vi "Configure Polarity.vi"(6 "channel (1)":i32=1 min=1 max=4, 8 "error in (no error)":errorcluster, 10 "Polarity (0: Positive)":T1 items=["Positive", "Negative"], 11 "VISA resource name":refnum<visa-resource-name>) -> (0 "error out":errorcluster, 3 "VISA resource name out":refnum<visa-resource-name>)   [LabVIEW 2019, in "Pulse Rider PG-1000.lvlib"]
doc: "This command set the output polarity.\n\npolarity: the polarity: 'positive' or 'negative'\nchannel: the output channel int from 1 to 4"
uses:
  <instrlib>/LV_PulseRiderPG1000/Pulse Rider PG-1000.lvlib
  <instrlib>/LV_PulseRiderPG1000/Public/Configure/Pulse/Polarity.ctl
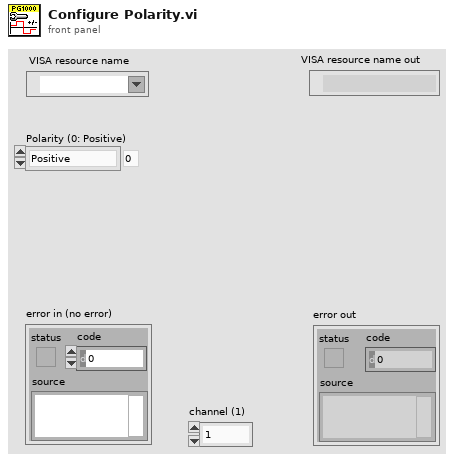
[diagram p1: front panel]
types:
  T1 = typedef "Pulse Rider PG-1000.lvlib/Polarity.ctl" = u16
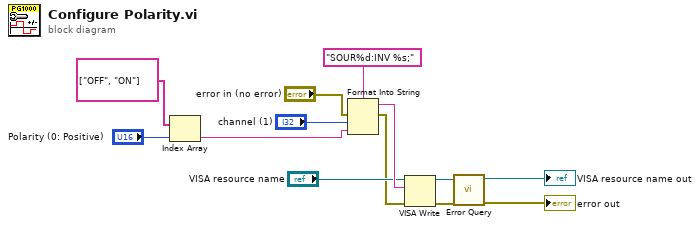
[diagram p0: block diagram]
diagram:
  n1 = Index Array(array=string[] ["OFF", "ON"], index="Polarity (0: Positive)") -> (element=w5:string)
  n2 = Format Into String(format string="SOUR%d:INV %s;", error in="error in (no error)", "channel (1)", w5) -> (resulting string=w10:string, error out=w2:errorcluster)  [unwired: 1 in]
  n3 = VISA Write(VISA resource name="VISA resource name", write buffer=w10, error in (no error)=w2) -> (VISA resource name out=w13:refnum<visa-resource-name>, error out=w12:errorcluster)  [unwired: 1 out]
  n4 = call <instrlib>:"Error Query.vi"("error in (no error)"=w12, "VISA resource name"=w13) -> ("error out"=→"error out":errorcluster, "VISA resource name out"=→"VISA resource name out":refnum<visa-resource-name>)  [unwired: 6 in, 2 out]
